vi "B_ReadProperty.vi"(8 "error in (no error)":errorcluster, 11 "reference in":refnum<class "BaseTemplate.lvclass">) -> (0 "error out":errorcluster, 2 "property":dbl, 3 "reference out":refnum<class "BaseTemplate.lvclass">)   [LabVIEW 2014, in "BaseTemplate.lvclass"]
uses:
  <resource>/Framework/Providers/Open_GDS/ClassProviders/Provider_EndevoGOOP300/Templates/BaseTemplate/BaseTemplate.lvclass
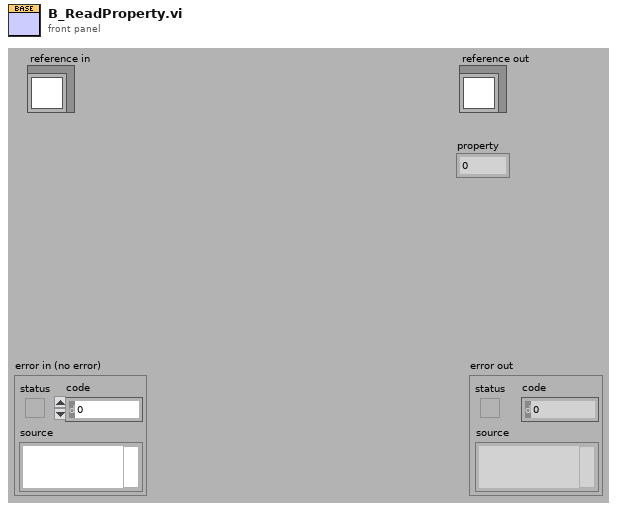
[diagram p1: front panel]
types:
  T1 = typedef "BaseTemplate.lvclass/ObjectAttributes.ctl" = cluster{"Attribute1":dbl}
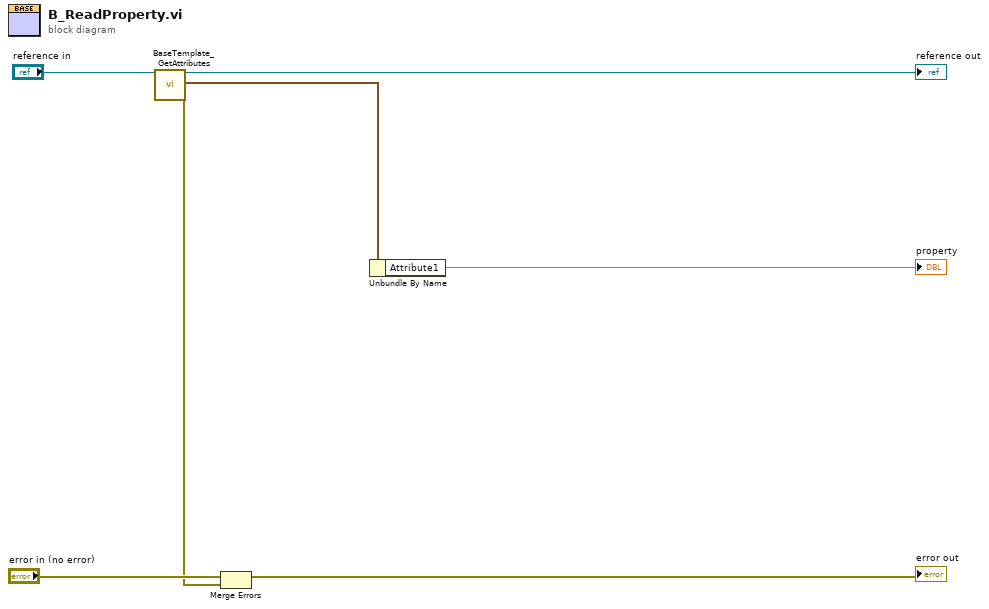
[diagram p0: block diagram]
diagram:
  n1 = call <resource>:"BaseTemplate_GetAttributes.vi"("reference in"="reference in") -> ("reference out"=→"reference out":refnum<class "BaseTemplate.lvclass">, "Attributes"=w4:T1, "error out"=w2:errorcluster)  [unwired: 15 in, 1 out]
  n2 = Merge Errors("error in (no error)", w2) -> (→"error out":errorcluster)
  n3 = Unbundle By Name(w4) -> ("Attribute1"=→"property":dbl)
